vi "State Check RSLinx Tag String 2.0.vi"(8 "Sys Error In":errorcluster, 9 "Main State Cluster":T1={"Application Status"="", "Switch Output Array"=[], "Switch Value Configuration"=[], "NVH Configuration"={"NVH Station?"=FALSE, "nvh app instance path"="", "NVH_ErrorMessages sv url"="", "NVH_Inputs sv url"="", "NVH_MotionNumber sv url"="", "NVH_Outputs sv url"="", "NVH_PartNumber sv url"="", "NVH_PartNumber_Echo sv url"="", "NVH_SerialNumber sv url"="", "NVH_AmbientTempF sv url"=""}, "rs232 port map"={"PMAC"="", "PS Port"="", "LVDT Unit"="", "RS232"=""}, "ethernet address map"={"LVDT 1 Unit"="172.17.53.143", "LVDT Unit 1 port"=0}, "paths"={"Base Path"=path "", "system error log path"=path "", "Error Table Path"=path "C/Labview Code/System/Error Table", "Store errors log path"=path "C/Labview Code/System/Error Table", "data bytes log path"=path "C/Labview Code/System/Error Table", "network path"=path "C/Labview Code/System/Error Table"}, "Station Index"=0, "Store Data"={"Motion Data Array"=[], "Error Table"=[], "Sun Shade Close Force Limits"={"Overall Min"=0.0, "Overall Max"=0.0, "Avg Min"=0.0, "Avg Max"=0.0, "Truncation Start"=0.0, "Truncation End"=0.0, "Variance"=0.0, "Check Noise"=FALSE}, "Sun Shade Open Force Limits"={"Overall Min"=0.0, "Overall Max"=0.0, "Avg Min"=0.0, "Avg Max"=0.0, "Truncation Start"=0.0, "Truncation End"=0.0, "Variance"=0.0, "Check Noise"=FALSE}, "Sunshade Open Data"=[], "Sunshade Close Data"=[], "Module Info"={"Serial Number"="", "Pallet Number"="", "Sunshade Color"="", "Inalfa Part Number"="", "Customer Number"=""}, "Sunsahde Close Raw Data"=[], "Sunshade Open Raw Data"=[], "Software Version"=[], "Constant Version"=[], "Hardware Version"=[], "Inalfa Part Number ECU"=[], "LVDT Data"=[], "Communication Line 1"=[], "Communication Line 2"=[], "Anti Pinch Force"=[], "Cycle Time"="", "Anti Pinch Vent Force"=[], "iGPS LVDT Data"=[], "data bytes log"=""}, "D in map"={"Abort Test"=enum."Dev2/port2/line6", "Start Test"=enum."Dev2/port2/line6"}, "DO Task"="", "ctl refs"={"Start Test"=refnum, "Abort Test"=refnum, "Manual Control"=refnum, "Route to Repair"=refnum, "Waveform Graph"=refnum, "Motion Data"=refnum, "all station status"=refnum, "Individual Station Status"=refnum, "exit program"=refnum, "Sunshade Servo Data Open"=refnum, "Sunshade Servo Data Close"=refnum, "Red-Rabbit Mode"=refnum, "Direct Manual Ctrl"=refnum}, "misc station config"={"Station Name"="", "is AT station?"=FALSE, "is audit station?"=FALSE, "power supply type"=enum."GENser", "use alt China TP2 LVDT Logic Seq"=FALSE, "hmi operator abort timeout"=0, "dump all analog values even if pass"=FALSE, "debug log pre-filter ap stream bytes"=FALSE, "use separate lvdt x and z extend tags"=FALSE, "is print"=FALSE}, "ethernet tcp refs"={"LVDT Unit"=refnum}, "Sunshade Barcode Scan"={"Sunshade Number 2"="", "Sunshade Number 1"="", "Keyence tuning bank idx"=0}, "AP Test Data"={"Raw Sunshade AP Data"="", "Raw Glass AP Data"="", "PMAC Read Counter"=0.0, "Database AP Data"=[]}, "Motion Status"={"hmi operator abort start time"=0, "Current Data Index"=0, "Analog Data"=[], "Motor Position Hex"=0, "Messages Index"=0, "Last Bytes"=[], "Current Hall Position"=0, "Motion Stop Timer"=0, "Position Test"=enum."Not Tested", "Noise Test"=enum."Not Tested", "motion stop check initialized"=FALSE, "remote sense enabled"=FALSE, "Motion"=enum."Glass Teach"}, "LVDT Status"={"LVDT's stored config"=[], "lvdt precision"={"truncate instead of rounding"=FALSE, "decimal places"=0}}, "Sequence State"={"Step Description"="", "Cycle Start Time"=0, "Step Data String"="", "Pass?"=FALSE, "Seqence"=[], "Active Step"=0, "Testing?"=FALSE, "Red-Rabbit Mode"=FALSE, "route-to-repair mode"=FALSE, "NVH Status"={"Restart IRQ Counter"=0, "NVH Test Needed?"=FALSE, "NVH Test Running?"=FALSE}, "Present (s)"=0.0, "Hold Mode?"=FALSE, "Hold?"=FALSE, "Rx Invalid?"=FALSE}, "misc status"={"delay start time (ticks)"=0, "In Vehicle Mode?"=FALSE, "Diag Mode?"=FALSE, "Serial Port Configured?"=FALSE, "PS Voltage"=0.0, "Diag Serial Port"="", "Part Setup"={"Communication Type"=enum."None", "Send Messages to"=enum."Glass", "RAP Signal"=enum."High", "Motor Type"=enum."Smart Motor", "NVH Part Number"=0, "Turn Off Timer"=0, "Part Type"=""}, "Part History Number"="", "Plant Number"=0, "AP Data Type"=enum."91/61", "Real Rollo?"=FALSE}, "NVH Operator?"=FALSE, "NVH Pass?"=FALSE, "Operator Pass?"=FALSE, "Operator Action?"=FALSE, "Noise Source"=0, "USBHandle"=0, "PeakInfo"="", "PeakNumber"=0, "NVH Motion Steps"=[], "Second Check?"=FALSE, "Decibel data"=[], "Direct Control Info"={"EnableStopOnHome"=FALSE, "EnableStopOnPos"=FALSE, "TeachEvent"=FALSE, "open offset"=0, "close offset"=0, "Derect control"=FALSE, "set position"=[], "teach pass "=FALSE, "Drift offsets"=[], "Hall Positions"=[]}, "manual control(direct)"=FALSE, "LIN INFO"={"Toolkit Type"=enum."Inalfa LIN", "NAD"=36, "Inalfa LIN"={"Master Frame(3C)"="", "Slave Frame(3D)"="NIXNET_exampleLDF", "Request Schedule"="NIXNET_exampleLDF", "Response Schedule"="CEMLIN3DiagResponseSchedule\nSPA3414_ConfigurationsCMAGeely_CEMCALYPSOSDB34XX0Cfg_LIN3_190709_", "Frame Write SCU"="", "Frame Read SCU"="", "LIN Name"=""}, "ADCS LIN"={"Port"="MasterReq\nSPA3414_ConfigurationsCMAGeely_CEMCALYPSOSDB34XX0Cfg_LIN3_190709_", "HW select"=0, "XNET Cluster"="SlaveResp\nSPA3414_ConfigurationsCMAGeely_CEMCALYPSOSDB34XX0Cfg_LIN3_190709_", "ByteCmd Path"=path "C/Labview Code/System/ByteCmdConfig.txt"}, "TS LIN"={"ref info"=refnum, "LIN Channel"=0, "ByteCmd Path"=path "C/Labview Code/System/ByteCmdConfig.txt"}}, "Config Info"=variant} {"LIN INFO"."NAD" format="%.0x"; "LIN INFO"."ADCS LIN"."HW select" items=["NI-XNET", "NI-CAN"]; "LVDT Status"."LVDT's stored config"."Lower Limit" format="%.2f"; "LVDT Status"."LVDT's stored config"."Upper Limit" format="%.2f"; "Store Data"."Sun Shade Open Force Limits"."Variance" format="%.2g"; "Store Data"."Sun Shade Open Force Limits"."Truncation End" format="%.2g"; "Store Data"."Sun Shade Open Force Limits"."Truncation Start" format="%.2g"; "Store Data"."Sun Shade Open Force Limits"."Avg Max" format="%.2g"; "Store Data"."Sun Shade Open Force Limits"."Avg Min" format="%.2g"; "Store Data"."Sun Shade Open Force Limits"."Overall Max" format="%.2g"; "Store Data"."Sun Shade Open Force Limits"."Overall Min" format="%.2g"; "Store Data"."Sun Shade Close Force Limits"."Variance" format="%.2g"; "Store Data"."Sun Shade Close Force Limits"."Truncation End" format="%.2g"; "Store Data"."Sun Shade Close Force Limits"."Truncation Start" format="%.2g"; "Store Data"."Sun Shade Close Force Limits"."Avg Max" format="%.2g"; "Store Data"."Sun Shade Close Force Limits"."Avg Min" format="%.2g"; "Store Data"."Sun Shade Close Force Limits"."Overall Max" format="%.2g"; "Store Data"."Sun Shade Close Force Limits"."Overall Min" format="%.2g"; "Store Data"."Motion Data Array"."Motion Data Limits"."LIN Msg"."Msg" format="%02x"; "Store Data"."Motion Data Array"."Motion Data Limits"."LIN Msg"."ID" format="%02x"}, 10 "Step Description":string, 11 "Step Data String":string) -> (0 "Sys Error Out":errorcluster, 1 "Error No.":u16, 2 "Error String":string, 3 "Pass?":bool)   [LabVIEW 2018]
uses:
  02.Type Def's/main state cluster.ctl
  02.Type Def's/All Switch Configuration Cluster.ctl
  02.Type Def's/All Motions.ctl
  02.Type Def's/EOL Switch Value Configuration Cluster.ctl
  02.Type Def's/EOL Switch Max Min Check Cluster.ctl
  02.Type Def's/station nvh config.ctl
  02.Type Def's/station rs232 port map.ctl
  02.Type Def's/station ethernet address map.ctl
  02.Type Def's/station paths.ctl
  02.Type Def's/EOL Save Module Test Data Control.ctl
  02.Type Def's/EOL Motion Database Table.ctl
  05.UserVI's/type defs/17x Audit Motion Data Seq Control.ctl
  05.UserVI's/type defs/17x AP Data Type.ctl
  05.UserVI's/type defs/17x Sunshade Limts Seq.ctl
  02.Type Def's/EOL Module Info Control.ctl
  02.Type Def's/station DI map.ctl
  05.UserVI's/type defs/EOL Global Digital Input Control.ctl
  02.Type Def's/control refs.ctl
  02.Type Def's/station motion data indicator.ctl
  02.Type Def's/Screen Motion Data.ctl
  02.Type Def's/Pass Fail Control.ctl
  02.Type Def's/station hmi.ctl
  02.Type Def's/lvdt name val pair.ctl
  02.Type Def's/individual station status.ctl
  02.Type Def's/misc station config.ctl
  05.UserVI's/Lambda Power/power supply types.ctl
  05.UserVI's/type defs/EOL LVDT's Check Controller.ctl
  05.UserVI's/LVDT's/lvdt precision.ctl
  02.Type Def's/sequence state.ctl
  05.UserVI's/sequence/type defs/Sequence Info.ctl
  05.UserVI's/type defs/EOL Part Setup.ctl
  02.Type Def's/All Communication Types.ctl
  05.UserVI's/type defs/Communication with Motors.ctl
  05.UserVI's/type defs/RAP Signal Control.ctl
  05.UserVI's/type defs/EOL Motor Type.ctl
  02.Type Def's/station LIN config.ctl
  03.Inalfa LIN/LIN Device.ctl
  <vilib>/CMC.AME/Inalfa ADCS/Ctl'Def/ADCS_LIN info.ctl
  C:/Program Files (x86)/National Instruments/LabVIEW 2018/vi.lib/CMC.AME/Inalfa TS LIN/TOSUN/TSMaster/bin/Interop.TSMasterAPI.dll
  Program Files (x86)/National Instruments/LabVIEW 2018/vi.lib/CMC.AME/Inalfa TS LIN/TOSUN/TSMaster/bin/Interop.TSMasterAPI.dll
  06.Test Loop/Sub'VIs/Type Def's/Config Info.ctl
panel:
  # "Sunroof Barcode"
  # "Pallet Number"
  # "Part Type"
  # "Application Status"
  # "Current Step"
  # "Cycle Time"
  # "Pass / Fail"
  # "Shade Close"
  # "Actual Data"
  # "Limits"
  # "Avg Current"
  # "Run Time"
  # "Speed"
  # "Noise Test"
  # "Position"
  # "Shade Open"
  # "Actual Data"
  # "Limits"
  # "Avg Current"
  # "Run Time"
  # "Speed"
  # "Noise Test"
  # "Position"
  # "Vent Close"
  # "Actual Data"
  # "Limits"
  # "Avg Current"
  # "Run Time"
  # "Speed"
  # "Noise Test"
  # "Position"
  # "Vent Open"
  # "Actual Data"
  # "Limits"
  # "Avg Current"
  # "Run Time"
  # "Speed"
  # "Noise Test"
  # "Position"
  # "Slide Close"
  # "Actual Data"
  # "Limits"
  # "Avg Current"
  # "Run Time"
  # "Speed"
  # "Noise Test"
  # "Position"
  # "Slide Open"
  # "Actual Data"
  # "Limits"
  # "Avg Current"
  # "Run Time"
  # "Speed"
  # "Noise Test"
  # "Position"
  # "Min"
  # "N"
  # "Min"
  # "Start"
  # "N"
  # "Max"
  # "N"
  # "Max"
  # "N"
  # "End"
  # "Min"
  # "N"
  # "Min"
  # "Start"
  # "N"
  # "Max"
  # "N"
  # "Max"
  # "N"
  # "End"
  # "Min"
  # "Max"
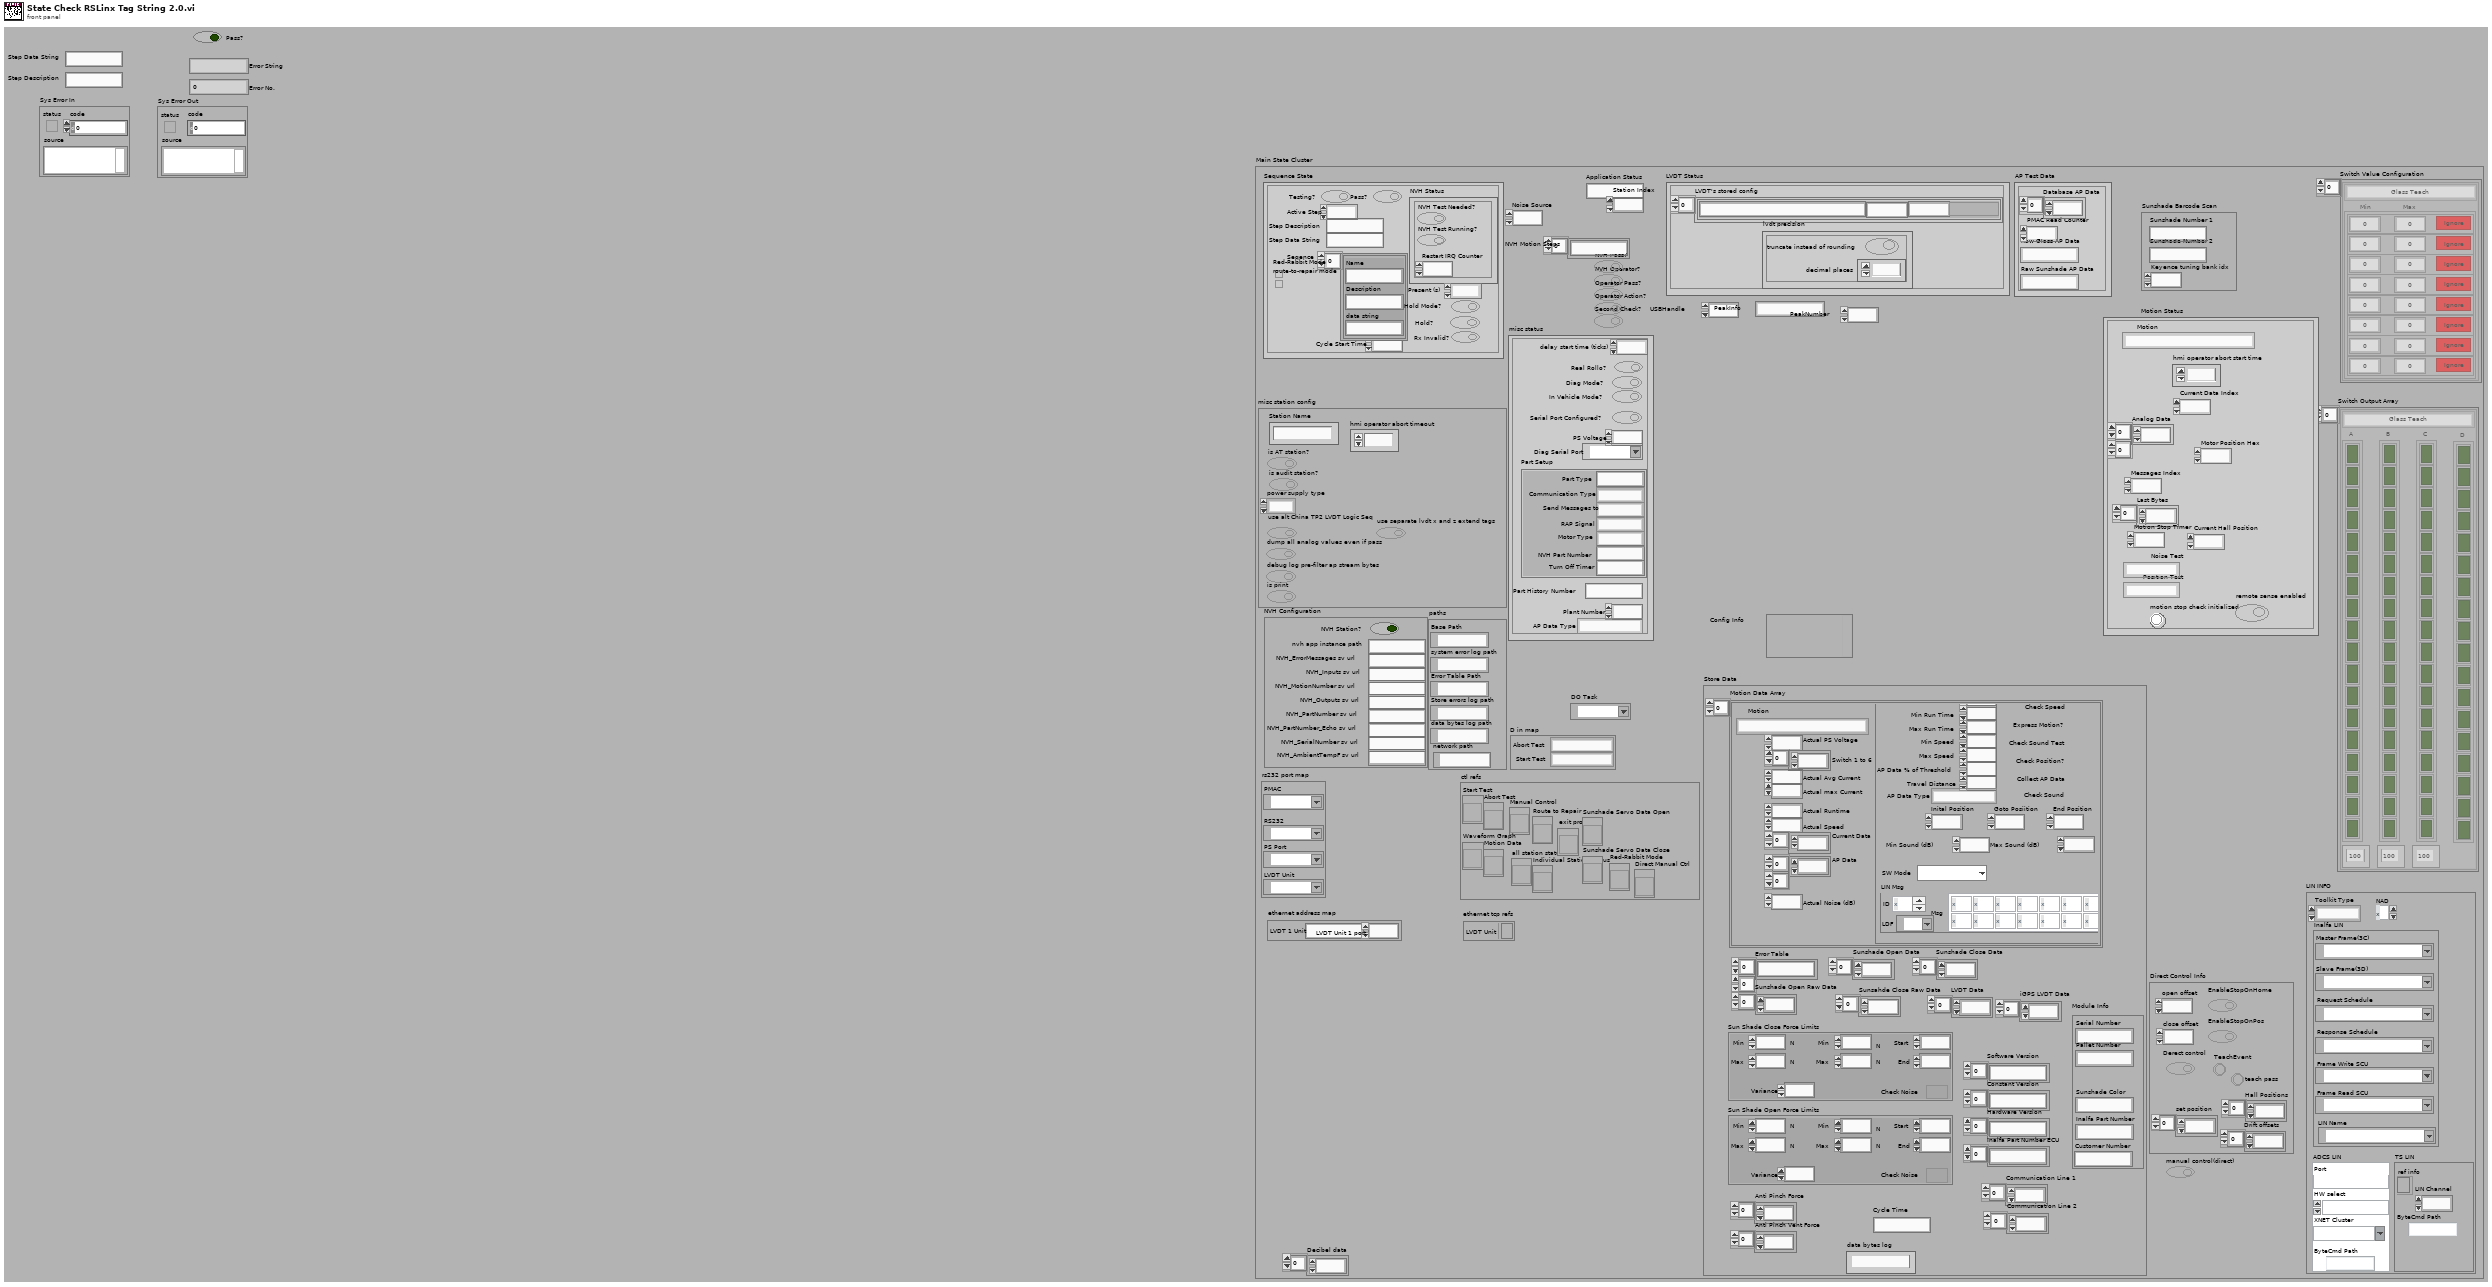
[diagram p1: front panel]
types:
  T1 = typedef "main state cluster.ctl" = cluster{"Application Status":string, "Switch Output Array":T2[], "Switch Value Configuration":T4[], "NVH Configuration":T6, "rs232 port map":T7, "ethernet address map":T8, "paths":T9, "Station Index":i32, "Store Data":T10, "D in map":T16, "DO Task":refnum<k21>, "ctl refs":T18, "misc station config":T19, "ethernet tcp refs":cluster{"LVDT Unit":refnum<k5>}, "Sunshade Barcode Scan":cluster{"Sunshade Number 2":string, "Sunshade Number 1":string, "Keyence tuning bank idx":i32}, "AP Test Data":cluster{"Raw Sunshade AP Data":string, "Raw Glass AP Data":string, "PMAC Read Counter":dbl, "Database AP Data":dbl[]}, "Motion Status":cluster{"hmi operator abort start time":u32, "Current Data Index":i32, "Analog Data":sgl[][], "Motor Position Hex":u16, "Messages Index":u16, "Last Bytes":u8[], "Current Hall Position":i16, "Motion Stop Timer":u32, "Position Test":T21, "Noise Test":T21, "motion stop check initialized":bool, "remote sense enabled":bool, "Motion":T3}, "LVDT Status":cluster{"LVDT's stored config":T22[], "lvdt precision":T23}, "Sequence State":T24, "misc status":cluster{"delay start time (ticks)":u32, "In Vehicle Mode?":bool, "Diag Mode?":bool, "Serial Port Configured?":bool, "PS Voltage":dbl, "Diag Serial Port":refnum<visa-resource-name>, "Part Setup":T26, "Part History Number":string, "Plant Number":u8, "AP Data Type":T13, "Real Rollo?":bool}, "NVH Operator?":bool, "NVH Pass?":bool, "Operator Pass?":bool, "Operator Action?":bool, "Noise Source":u32, "USBHandle":i32, "PeakInfo":string, "PeakNumber":i32, "NVH Motion Steps":string[], "Second Check?":bool, "Decibel data":dbl[], "Direct Control Info":cluster{"EnableStopOnHome":bool, "EnableStopOnPos":bool, "TeachEvent":bool, "open offset":i32, "close offset":i32, "Derect control":bool, "set position":i32[], "teach pass ":bool, "Drift offsets":i32[], "Hall Positions":i32[]}, "manual control(direct)":bool, "LIN INFO":T31, "Config Info":T34}
  T2 = typedef "All Switch Configuration Cluster.ctl" = cluster{"All Motions":T3, "A":bool[], "B":bool[], "C":bool[], "D":bool[], "A activation time (ms)":u32, "B activation time (ms)":u32, "C activation time (ms)":u32}
  T3 = typedef "All Motions.ctl" = enum16{"Glass Teach", "Glass Slide Open", "Glass Slide Close", "Glass Vent Open", "Glass Vent Close", "Sunshade Teach", "Sunshade Open", "Sunshade Close", "Idle", "Sunshade Open 2", "Sunshade Close 2", "Glass Slide Open Sunshade Open", "Glass Slide Open Sunshade Close", "Glass Slide Close Sunshade Open", "Glass Slide Close Sunshade Close", "Glass Vent Open Sunshade Open", "Glass Vent Open Sunshade Close", "Glass Vent Close Sunshade Open", "Glass Vent Close Sunshade Close", "Express Glass Slide Open", "Express Glass Slide Close", "Express Glass Vent Open", "Express Glass Vent Close", "Express Sunshade Open", "Express Sunshade Close", "Express Sunshade Open 2", "Express Sunshade Close 2", "Express Glass Slide Open Sunshade Open", "Express Glass Slide Open Sunshade Close", "Express Glass Slide Close Sunshade Open", "Express Glass Slide Close Sunshade Close", "Express Glass Vent Open Sunshade Open", "Express Glass Vent Open Sunshade Close", "Express Glass Vent Close Sunshade Open", "Express Glass Vent Close Sunshade Close", "Goto Position Glass", "Goto Position Sunshade", "Sunshade Teach 2"}
  T4 = typedef "EOL Switch Value Configuration Cluster.ctl" = cluster{"All Motions":T3, "Array":T5[]}
  T5 = typedef "EOL Switch Max Min Check Cluster.ctl" = cluster{"Min":dbl, "Max":dbl, "Check?":bool}
  T6 = typedef "station nvh config.ctl" = cluster{"NVH Station?":bool, "nvh app instance path":string, "NVH_ErrorMessages sv url":string, "NVH_Inputs sv url":string, "NVH_MotionNumber sv url":string, "NVH_Outputs sv url":string, "NVH_PartNumber sv url":string, "NVH_PartNumber_Echo sv url":string, "NVH_SerialNumber sv url":string, "NVH_AmbientTempF sv url":string}
  T7 = typedef "station rs232 port map.ctl" = cluster{"PMAC":refnum<visa-resource-name>, "PS Port":refnum<visa-resource-name>, "LVDT Unit":refnum<visa-resource-name>, "RS232":refnum<visa-resource-name>}
  T8 = typedef "station ethernet address map.ctl" = cluster{"LVDT 1 Unit":string, "LVDT Unit 1 port":u16}
  T9 = typedef "station paths.ctl" = cluster{"Base Path":path, "system error log path":path, "Error Table Path":path, "Store errors log path":path, "data bytes log path":path, "network path":path}
  T10 = typedef "EOL Save Module Test Data Control.ctl" = cluster{"Motion Data Array":T11[], "Error Table":string[][], "Sun Shade Close Force Limits":T14, "Sun Shade Open Force Limits":T14, "Sunshade Open Data":sgl[], "Sunshade Close Data":sgl[], "Module Info":T15, "Sunsahde Close Raw Data":sgl[], "Sunshade Open Raw Data":sgl[], "Software Version":string[], "Constant Version":string[], "Hardware Version":string[], "Inalfa Part Number ECU":string[], "LVDT Data":sgl[], "Communication Line 1":sgl[], "Communication Line 2":sgl[], "Anti Pinch Force":sgl[], "Cycle Time":string, "Anti Pinch Vent Force":sgl[], "iGPS LVDT Data":sgl[], "data bytes log":string}
  T11 = typedef "EOL Motion Database Table.ctl" = cluster{"Motion":T3, "Actual Avg Current":dbl, "Actual Runtime":dbl, "Actual Speed":dbl, "Current Data":sgl[], "Motion Data Limits":T12, "Switch 1 to 6":dbl[], "Actual PS Voltage":dbl, "AP Data":i16[][], "Actual max Current":dbl, "Actual Noise (dB)":dbl}
  T12 = typedef "17x Audit Motion Data Seq Control.ctl" = cluster{"Power Supply Voltage":dbl, "Min Avg Current":dbl, "Max Avg Current":dbl, "Min Run Time":dbl, "Max Run Time":dbl, "Min Speed":dbl, "Max Speed":dbl, "AP Data % of Threshold":dbl, "Travel Distance":dbl, "AP Data Type":T13, "Check Current":bool, "Check Run Time":bool, "Check Speed":bool, "Express Motion?":bool, "Check Sound Test":bool, "Check Position?":bool, "Collect AP Data":bool, "Inital Position":u16, "End Position":u16, "Goto Posiition":u16, "Max max Current":dbl, "Min max Current":dbl, "Check max Current":bool, "Check Sound":bool, "Min Sound (dB)":dbl, "Max Sound (dB)":dbl, "SW Mode":enum16{"Hard Switch", "Uncond Frame"}, "LIN Msg":cluster{"ID":u8, "Msg":u8[][], "LDF":refnum<k21>}}
  T13 = typedef "17x AP Data Type.ctl" = enum16{"91/61", "92/62", "93/63", "67", "68", "6F", "71", "91 Msg", "92 Msg", "93 Msg", "94 Msg", "HiRain 91", "HiRain 92 Speed", "HiRain 92 HS", "HiRain 92", "HiRain 93", "SnT"}
  T14 = typedef "17x Sunshade Limts Seq.ctl" = cluster{"Overall Min":dbl, "Overall Max":dbl, "Avg Min":dbl, "Avg Max":dbl, "Truncation Start":dbl, "Truncation End":dbl, "Variance":dbl, "Check Noise":bool}
  T15 = typedef "EOL Module Info Control.ctl" = cluster{"Serial Number":string, "Pallet Number":string, "Sunshade Color":string, "Inalfa Part Number":string, "Customer Number":string}
  T16 = typedef "station DI map.ctl" = cluster{"Abort Test":T17, "Start Test":T17}
  T17 = typedef "EOL Global Digital Input Control.ctl" = enum16{"Dev2/port0/line0", "Dev2/port0/line1", "Dev2/port0/line2", "Dev2/port0/line3", "Dev2/port0/line4", "Dev2/port0/line5", "Dev2/port0/line6", "Dev2/port0/line7", "Dev2/port1/line0", "Dev2/port1/line1", "Dev2/port1/line2", "Dev2/port1/line3", "Dev2/port1/line4", "Dev2/port1/line5", "Dev2/port1/line6", "Dev2/port1/line7", "Dev2/port2/line0", "Dev2/port2/line1", "Dev2/port2/line2", "Dev2/port2/line3", "Dev2/port2/line4", "Dev2/port2/line5", "Dev2/port2/line6", "Dev2/port2/line7", "Prerun Start Test", "Prerun Abort Test", "Audit Start Test", "Audit Abort Test", "Dev2/port3/line4", "Dev2/port3/line5", "Breakin Start Test", "Breakin Abort Test", "Not Implemented"}
  T18 = typedef "control refs.ctl" = cluster{"Start Test":refnum<vi>, "Abort Test":refnum<vi>, "Manual Control":refnum<vi>, "Route to Repair":refnum<vi>, "Waveform Graph":refnum<vi>, "Motion Data":refnum<vi>, "all station status":refnum<vi>, "Individual Station Status":refnum<vi>, "exit program":refnum<vi>, "Sunshade Servo Data Open":refnum<vi>, "Sunshade Servo Data Close":refnum<vi>, "Red-Rabbit Mode":refnum<vi>, "Direct Manual Ctrl":refnum<vi>}
  T19 = typedef "misc station config.ctl" = cluster{"Station Name":string, "is AT station?":bool, "is audit station?":bool, "power supply type":T20, "use alt China TP2 LVDT Logic Seq":bool, "hmi operator abort timeout":u32, "dump all analog values even if pass":bool, "debug log pre-filter ap stream bytes":bool, "use separate lvdt x and z extend tags":bool, "is print":bool}
  T20 = typedef "power supply types.ctl" = enum16{"GENser", "ZUPser", "GENeth", "Manual", "ITECH"}
  T21 = typedef "Pass Fail Control.ctl" = enum16{"Not Tested", "Pass", "Fail"}
  T22 = typedef "EOL LVDT's Check Controller.ctl" = cluster{"Upper Limit":dbl, "Lower Limit":dbl, "LVDT Name":string, "Check":bool}
  T23 = typedef "lvdt precision.ctl" = cluster{"truncate instead of rounding":bool, "decimal places":u8}
  T24 = typedef "sequence state.ctl" = cluster{"Step Description":string, "Cycle Start Time":u32, "Step Data String":string, "Pass?":bool, "Seqence":T25[], "Active Step":u8, "Testing?":bool, "Red-Rabbit Mode":bool, "route-to-repair mode":bool, "NVH Status":cluster{"Restart IRQ Counter":u8, "NVH Test Needed?":bool, "NVH Test Running?":bool}, "Present (s)":dbl, "Hold Mode?":bool, "Hold?":bool, "Rx Invalid?":bool}
  T25 = typedef "Sequence Info.ctl" = cluster{"Name":string, "Description":string, "data string":string}
  T26 = typedef "EOL Part Setup.ctl" = cluster{"Communication Type":T27, "Send Messages to":T28, "RAP Signal":T29, "Motor Type":T30, "NVH Part Number":u16, "Turn Off Timer":u16, "Part Type":string}
  T27 = typedef "All Communication Types.ctl" = enum16{"None", "CAN", "RS 232", "RS 232 LIN", "GM LIN", "SnT LIN", "K Line", "Robel CAN", "P42M-Continental", "Inalfa SCU LIN", "Spare 3"}
  T28 = typedef "Communication with Motors.ctl" = enum16{"Glass", "Rollo", "Both"}
  T29 = typedef "RAP Signal Control.ctl" = enum16{"High", "Low", "None"}
  T30 = typedef "EOL Motor Type.ctl" = enum16{"Smart Motor", "Sensor Motor"}
  T31 = typedef "station LIN config.ctl" = cluster{"Toolkit Type":enum16{"Inalfa LIN", "ADCS LIN", "TS LIN"}, "NAD":u8, "Inalfa LIN":T32, "ADCS LIN":T33, "TS LIN":cluster{"ref info":refnum<k24>, "LIN Channel":i32, "ByteCmd Path":path}}
  T32 = typedef "LIN Device.ctl" = cluster{"Master Frame(3C)":refnum<k21>, "Slave Frame(3D)":refnum<k21>, "Request Schedule":refnum<k21>, "Response Schedule":refnum<k21>, "Frame Write SCU":refnum<k21>, "Frame Read SCU":refnum<k21>, "LIN Name":refnum<k21>}
  T33 = typedef "ADCS_LIN info.ctl" = cluster{"Port":string, "HW select":u16, "XNET Cluster":string, "ByteCmd Path":path}
  T34 = typedef "Config Info.ctl" = variant
  T35 = typedef "plc comms params.ctl" = cluster{"PLC boolean read Tags":T36, "PLC bool write Tags":T39, "PLC string read Tags":T40, "PLC string write Tags":T41, "use opc":bool, "PLC/OPC Path":string}
  T36 = typedef "station plc read boolean tags.ctl" = cluster{"AT glass position":T37, "AT shade position":T37, "AT in glass wand lower pos":T37, "AT in glass wand up pos":T37, "AT in sunshad wand lower pos":T37, "AT in sunshad wand up pos":T37, "AT in wand home pos":T37, "LVDT's Extended":T37, "bolt check 1":T37, "bolt check 2":T37, "bolt check 3":T37, "bolt check 4":T37, "bolt check 5":T37, "bolt check 6":T37, "bolt check 7":T37, "bolt check 8":T37, "start":T37, "abort":T37, "LVDT's Retracted":T37, "manual barcode print":T37, "ss servo at open":T37, "ss servo at close":T37, "ss servo opening":T37, "ss servo closing":T37, "control slide at home":T37, "control slide left good":T37, "control slide left over stroke":T37, "control slide right good":T37, "control slide right over stroke":T37, "wind deflector high speed pos":T37, "wind deflector low speed pos":T37, "AT VentPMACatHome":T37, "AT VentPMACisExtend":T37, "SS Barcode Scanner Bypassed":T37, "Check Frame Barcode":T37, "Z LVDTs Extended":T37, "NVH Operator Pass":T37, "NVH Operator Fail":T37, "NVH Operator Express Glass Open":T37, "NVH Operator Express Glass Close":T37, "NVH Operator Express Rollo Open01":T37, "NVH Operator Express Rollo Close01":T37, "NVH Operator Express Rollo Open02":T37, "NVH Operator Express Rollo Close02":T37, "NVH Operator Vent Open Noise":T37, "NVH Operator Vent Close Noise":T37, "NVH Operator Sunshade Open Noise":T37, "NVH Operator Sunshade Close Noise":T37, "NVH Operator Glass Open Noise":T37, "NVH Operator Glass Close Noise":T37, "NVH Operator Finish":T37, "NVH Operator Check":T37, "windproof position":T37, "NVH Operator Express Glass vent Open":T37, "NVH Operator Express Glass Vent Close":T37, "NVH Operator Re-do":T37, "AT at vent ATS test pos":T37, "AT at vent ATS Home pos":T37, "Start Adjust LVDT":T37, "Finish Adjust LVDT":T37}
  T37 = typedef "plc path and tag.ctl" = cluster{"Tag Name":string, "Network Path":string, "use opc":bool, "DataSocket Reference":T38}
  T38 = typedef "DataSocket Reference Type.ctl" = cluster{"CWDSLib._DCWDataSocket":refnum<k7>, "CWDSLib._DCWData":refnum<k7>, "OnDataUpdated":u32, "OnStatusUpdated":u32}
  T39 = typedef "station plc write boolean tags.ctl" = cluster{"AT set glass wand lower":T37, "AT set sunshade wand lower":T37, "AT set sunshade wand up":T37, "AT set glass wand up":T37, "AT set wand home pos":T37, "Test Complete Pass":T37, "Test Complete Fail":T37, "Test Started":T37, "Retract LVDT's":T37, "Extend LVDT's":T37, "ss servo open":T37, "ss servo close":T37, "control slide start":T37, "control slide stop":T37, "AT VentPMACHome":T37, "AT VentPMACExtended":T37, "Good Frame Barcode":T37, "Bad Frame Barcode":T37, "Extend Z LVDTS":T37, "NVH SunRoof Moving":T37, "NVH SunRoof Stop":T37, "NVH Pass":T37, "NVH Fail":T37, "NVH Operator Express Glass Opened":T37, "NVH Operator Express Glass Closed":T37, "NVH Operator Express Rollo Opened01":T37, "NVH Operator Express Rollo Closed01":T37, "NVH Operator Express Rollo Opened02":T37, "NVH Operator Pass":T37, "NVH Operator Fail":T37, "NVH Operator Check":T37, "NVH Operator Vent Open Noise":T37, "NVH Operator Vent Close Noise":T37, "NVH Operator Sunshade Open Noise":T37, "NVH Operator Sunshade Close Noise":T37, "NVH Operator Glass Open Noise":T37, "NVH Operator Glass Close Noise":T37, "NVH Operator Finish":T37, "Barcode01 OK":T37, "Barcode02 OK":T37, "AT set to Vent ATS Test Pos":T37, "AT set to Vent ATS Home Pos":T37, "Move LVDT Adjust Station":T37}
  T40 = typedef "station plc read string tags.ctl" = cluster{"Serial Number":T37, "Pallet Number":T37, "Inalfa Part Number":T37, "Shade Color":T37, "Model Type":T37, "Customer Number":T37, "Part History Number":T37, "Shade 1 Barcode":T37, "Shade 2 Barcode":T37, "Manual Serial Number":T37, "Manual Inalfa Part Number":T37, "Manual Shade Color":T37, "Manual Model Type":T37, "Manual Customer Number":T37, "Manual Part History Number":T37}
  T41 = typedef "station plc write string tags.ctl" = cluster{"barcode station error":T37, "error message 0":T37, "error message 1":T37, "error message 2":T37, "error message 3":T37}
  T42 = typedef "RSLinx String Cluster.ctl" = cluster{"Data String":string, "PLC Path and Tag":T37, "Error No.":u16, "timeout (ms)":i32}
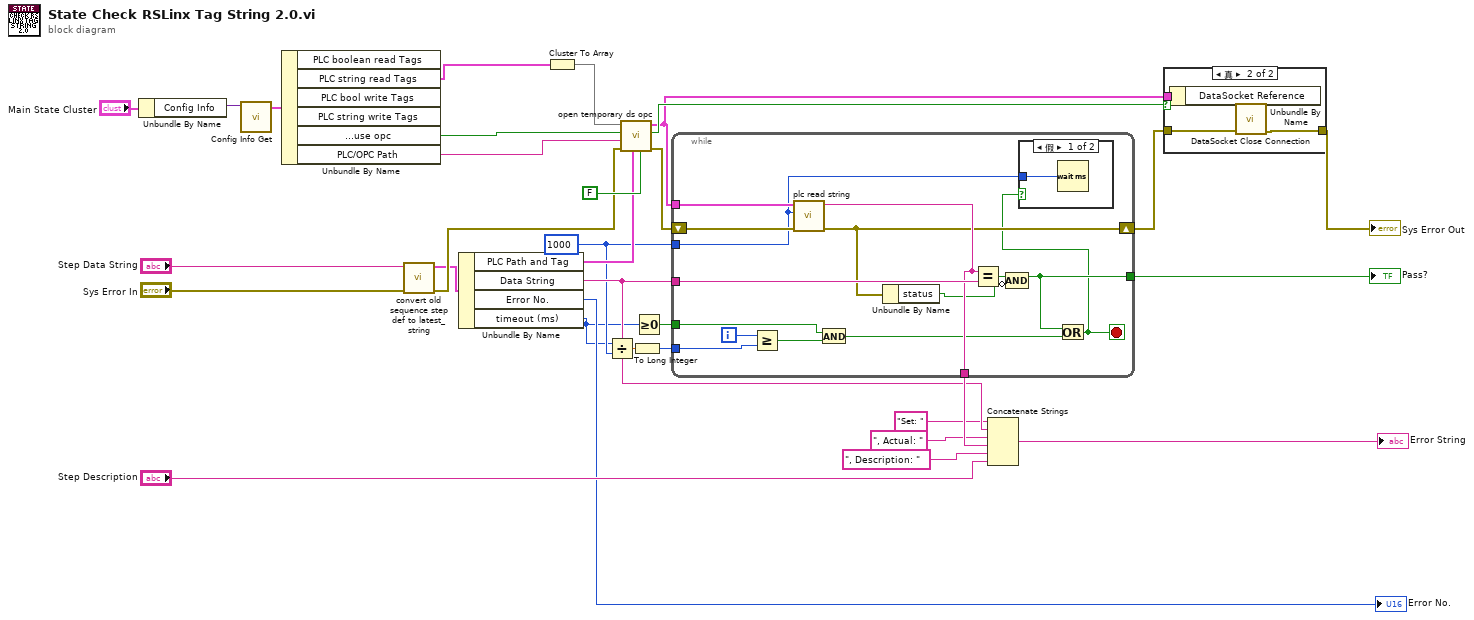
[diagram p0: block diagram]
diagram:
  w7 = 1000 ("milliseconds to wait")
  n1 = Unbundle By Name("Main State Cluster") -> ("Config Info"=w2:T34)
  n2 = call "Config Info Get.vi"("Config Info"=w2) -> ("PLC Comms"=w1:T35)  [unwired: 7 in, 3 out]
  n3 = Unbundle By Name(w1) -> ("PLC string read Tags"=w17:T40, "PLC boolean read Tags.AT glass position.use opc"=w24:bool, "PLC/OPC Path"=w23:string)  [unwired: 3 out]
  n4 = call "convert old sequence step def to latest_string.vi"("error in"="Sys Error In", "data string"="Step Data String") -> ("error out"=w11:errorcluster, "RSLinx String Cluster out"=w9:T42)  [unwired: 8 in]
  n5 = Unbundle By Name(w9) -> ("PLC Path and Tag"=w16:T37, "Data String"=w27:string, "Error No."=→"Error No.":u16, "timeout (ms)"=w5:i32)
  n6 = Cluster To Array(cluster=w17) -> (array=w22:T37[])
  n7 = Divide(x=w5, y=w7) -> (x/y=w8:dbl)
  n8 = call "open temporary ds opc.vi"("read=f,write=t"=FALSE, "PLC Path and Tag in"=w16, "error in"=w11, "PLC/OPC Path"=w23, "use opc"=w24, "PLC boolean read Tags"=w22) -> ("error out"=w20:errorcluster, "close ds after io"=w15:bool, "PLC Path and Tag out"=w14:T37)  [unwired: 3 in]
  n9 = To Long Integer(number=w8) -> (32bit integer=w6:i32)
  n10 = Greater Or Equal To 0?(x=w5) -> (x >= 0?=w4:bool)
  n11 = while {
    tunnel: [w42] -> w29
    tunnel: w27 -> [w47]
    tunnel: [w41] -> w25
    tunnel: w14 -> [w44]
    shift-right: [w40] -> w19
    shift-left: w20 -> [w43]
    tunnel: w7 -> [w37]
    tunnel: w6 -> [w36]
    tunnel: w4 -> [w33]
    i -> [w45]
    stop <- w38 stop-if-true
    n12 = Greater Or Equal?(x=w45, y=w36) -> (x >= y?=w34:bool)
    n13 = call "plc read string.vi"("error in"=w43, "Timeout (ms)"=w37, "addr,tag"=w44) -> ("error out"=w40:errorcluster, "Data"=w42:string)  [unwired: 7 in]
    n14 = And(x=w33, y=w34) -> (x .and. y?=w35:bool)
    n15 = Unbundle By Name(w40) -> ("status"=w39:bool)
    n16 = Equal?(x=w42, y=w47) -> (x = y?=w46:bool)
    n17 = Compound Arithmetic op=AND(w46, invert w39) -> (w41:bool)
    n18 = Or(x=w41, y=w35) -> (x .or. y?=w38:bool)
    n19 = case shown="假" w38 {
      tunnel: w37 -> [w48 _]
      frame False {
        n20 = Wait (ms)(milliseconds to wait=w48) -> ()  [unwired: 1 out]
      }
      frame True {
      }
    }
  }
  "Pass?" <- w25
  n21 = Concatenate Strings("Set: " ("string"), w27, ", Actual: " ("string"), w29, ", Description: " ("string"), "Step Description") -> (→"Error String":string)
  n22 = case shown="真" w15 {
    tunnel: w19 -> [w49 w53]
    tunnel: [w49 w52] -> w18
    tunnel: w14 -> [_ w51]
    frame False {
    }
    frame True {
      n23 = Unbundle By Name(w51) -> ("DataSocket Reference"=w50:T38)
      n24 = call <vilib>:"DataSocket Close Connection.vi"("error in (no error)"=w53, "DataSocket Reference In"=w50) -> ("error out"=w52:errorcluster)  [unwired: 7 in]
    }
  }
  "Sys Error Out" <- w18
